vi "Execute.RunStimulus.vi"(8 "error in (no error)":errorcluster, 11 "Cluster":T1) -> (0 "error out":errorcluster)   [LabVIEW 2013, in "Simple Sequence Editor.lvlib"]
uses:
  Simple Sequence Editor.lvlib
  Types/Execuction.StateVariables.ctl
  <vilib>/NI Veristand/Execution/SequenceExecutionInterface/Stimulus Profile Session Ref.ctl
  NationalInstruments.VeriStand.ClientAPI
  <vilib>/NI Veristand/Execution/Workspace/SystemStateRegEventRef.ctl
  <vilib>/NI Veristand/Execution/Workspace/SystemStateEventRef.ctl
  <vilib>/NI Veristand/Execution/Workspace/WorkspaceAPI.ctl
  <vilib>/NI Veristand/Execution/SequenceExecutionInterface/Sequence Input Assignment Ref.ctl
  <vilib>/NI Veristand/Execution/SequenceExecutionInterface/NI_VS Sequence Execution Interface.lvlib
  <vilib>/NI Veristand/Execution/Workspace/NI_VS Workspace ExecutionAPI.lvlib
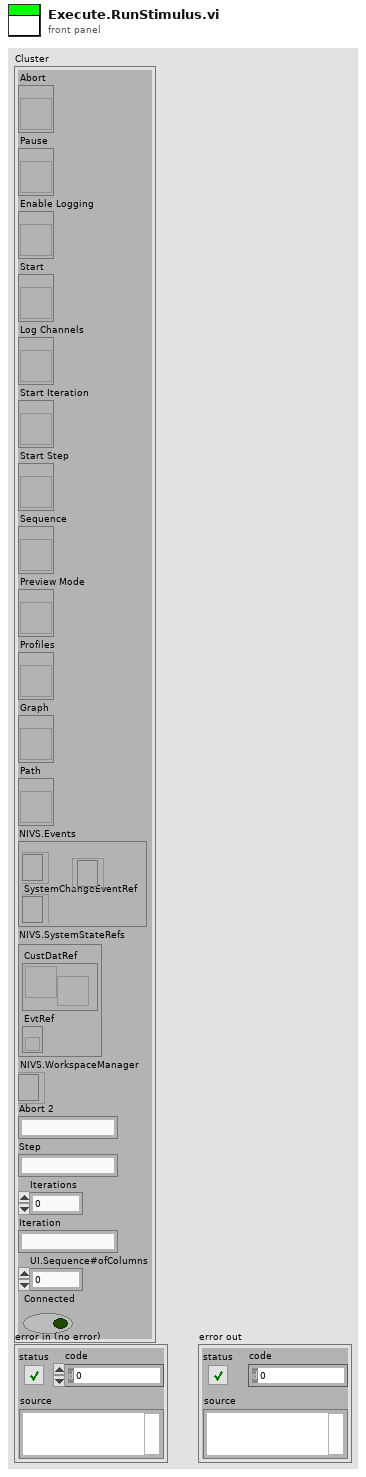
[diagram p1: front panel]
types:
  T1 = typedef "Simple Sequence Editor.lvlib/Execuction.StateVariables.ctl" = cluster{"Abort":refnum<vi>, "Pause":refnum<vi>, "Enable Logging":refnum<vi>, "Start":refnum<vi>, "Log Channels":refnum<vi>, "Start Iteration":refnum<vi>, "Start Step":refnum<vi>, "Sequence":refnum<vi>, "Preview Mode":refnum<vi>, "Profiles":refnum<vi>, "Graph":refnum<vi>, "Path":refnum<vi>, "NIVS.Events":cluster{"Complete":refnum<event-registration>, "NIVS.Workspace Event":refnum<event-registration>, "SystemChangeEventRef":T2}, "NIVS.SystemStateRefs":T3, "NIVS.WorkspaceManager":T4, "Abort 2":string, "Step":string, "Iterations":u32, "Iteration":string, "UI.Sequence#ofColumns":i32, "Connected":bool}
  T2 = typedef "NI_VS Workspace ExecutionAPI.lvlib/SystemStateRegEventRef.ctl" = refnum<event-registration>
  T3 = typedef "NI_VS Workspace ExecutionAPI.lvlib/SystemStateEventRef.ctl" = cluster{"CustDatRef":refnum<user-event>, "EvtRef":refnum<k27>}
  T4 = typedef "NI_VS Workspace ExecutionAPI.lvlib/WorkspaceAPI.ctl" = refnum<k24>
  T5 = typedef "NI_VS Sequence Execution Interface.lvlib/Sequence Input Assignment Ref.ctl" = refnum<k24>
  T6 = typedef "NI_VS Sequence Execution Interface.lvlib/Sequence Call Ref.ctl" = refnum<k24>
  T7 = typedef "NI_VS Sequence Execution Interface.lvlib/Stimulus Profile Session Ref.ctl" = refnum<k24>
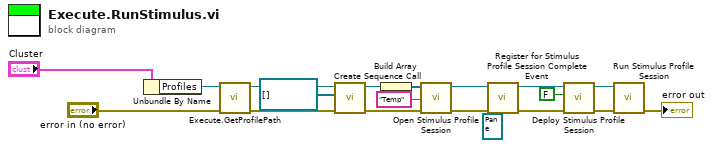
[diagram p0: block diagram]
diagram:
  (unwired) refnum<event-registration> refnum ("Event Registration Refnum")
  n1 = Unbundle By Name("Cluster") -> ("Profiles"=w18:refnum<vi>)
  n2 = call "Execute.GetProfilePath.vi"("error in (no error)"="error in (no error)", "Ring in"=w18) -> ("error out"=w3:errorcluster, "appended path"=w2:path)  [unwired: 8 in]
  n3 = call <vilib>:"Create Sequence Call.vi"("error in (no error)"=w3, "Parameter Assignments"=T5[] [], "Sequence File Path"=w2) -> ("error out"=w8:errorcluster, "Sequence Call Ref"=w7:T6)  [unwired: 7 in]
  n4 = Build Array(w7) -> (w10:T6[])
  n5 = call <vilib>:"Open Stimulus Profile Session.vi"("error in (no error)"=w8, "Session Name"="Temp", "Sequence Calls"=w10) -> ("error out"=w9:errorcluster, "Session Ref"=w11:T7)  [unwired: 7 in]
  n6 = call <vilib>:"Register for Stimulus Profile Session Complete Event.vi"("error in (no error)"=w9, "Session Ref in"=w11) -> ("error out"=w5:errorcluster, "Session Ref out"=w6:T7)  [unwired: 6 in, 2 out]
  n7 = call <vilib>:"Deploy Stimulus Profile Session.vi"("error in (no error)"=w5, "Auto-Start (T)"=FALSE, "Session Ref in"=w6) -> ("error out"=w14:errorcluster, "Session Ref out"=w13:T7)  [unwired: 6 in, 1 out]
  n8 = call <vilib>:"Run Stimulus Profile Session.vi"("error in (no error)"=w14, "Session Ref in"=w13) -> ("error out"=→"error out":errorcluster)  [unwired: 8 in, 1 out]
